vi "Disconnect from PIMHW Engine.vi"(6 "Legacy (f)?":bool, 8 "error in (no error)":errorcluster) -> (0 "error out":errorcluster)   [LabVIEW 2011]
uses:
  HW IO/HWIO Global.vi
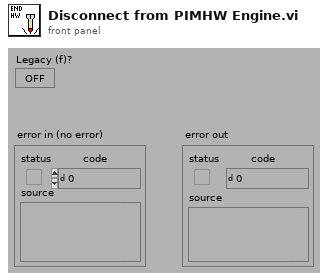
[diagram p1: front panel]
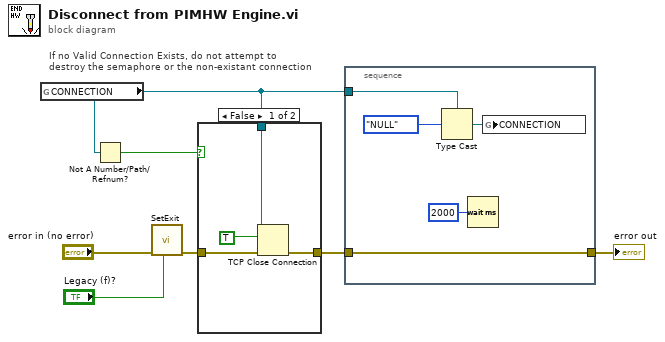
[diagram p0: block diagram]
diagram:
  # "If no Valid Connection Exists, do not attempt to\ndestroy the semaphore or the non-existant connection"
  n1 = global read "HWIO Global.vi" "CONNECTION"() -> (w4:refnum<k5>)
  n2 = Not A Number/Path/Refnum?(number/path/refnum=w4) -> (NaN/Path/Refnum?=w7:bool)
  n3 = call "SetExit.vi"("Legacy (f)?"="Legacy (f)?", "error in (no error)"="error in (no error)") -> ("error out"=w1:errorcluster)  [unwired: 9 out]
  n4 = case shown="False" w7 {
    tunnel: w1 -> [w8 w12]
    tunnel: [w11 w12] -> w6
    tunnel: w4 -> [w10 _]
    frame False {
      n5 = TCP Close Connection(connection ID=w10, abort (F)=TRUE, error in (no error)=w8) -> (error out=w11:errorcluster)  [unwired: 1 out]
    }
    frame True {
    }
  }
  n6 = stacked-sequence {
    tunnel: w6 -> [w17]
    tunnel: [w17] -> w5
    tunnel: w4 -> [w16]
    frame #0 {
      n7 = Type Cast(type=w16, x=enum16{"NULL"}."NULL") -> (*(type *) &x=w15:refnum<k5>)
      n8 = Wait (ms)(milliseconds to wait=u32 2000) -> ()  [unwired: 1 out]
      n9 = global write "HWIO Global.vi" "CONNECTION"(w15) -> ()
    }
  }
  "error out" <- w5
